vi "Request Multiple Data.vi"(4 "Ignore Past Updates? (F)":bool, 5 "Return Priority (Normal)":T2=enum."Normal", 6 "Value Changes Only? (T)":bool=TRUE, 7 "Activate Immediately? (T)":bool=TRUE, 8 "error in (no error)":errorcluster, 9 "Data Type":variant, 10 "Datum Names":string[](array[string]), 11 "IObserver in":refnum<class "IObserver.lvclass">) -> (0 "error out":errorcluster, 2 "Subscription Policies":T1[](array[typedef]), 3 "IObserver out":refnum<class "IObserver.lvclass">)   [LabVIEW 2015, in "IObserver.lvlib" / "IObserver.lvclass"]
doc: "<License>\nCopyright © 2017 Composed Systems, LLC | All rights reserved\nwww.composed.io\n\nAuthor: Ethan Stern <ethan.stern@composed.io>\n\nThis software is provided \"AS IS\" WITHOUT WARRANTIES, either express or implied, AND IS FOR EDUCATIONAL PURPOSES ONLY.\n</License>"
uses:
  IObserver.lvclass
  <vilib>/ActorFramework/Message Enqueuer/Message Priority.ctl
  IMediator/ISubscriptionPolicy/ISubscriptionPolicy Reference.ctl
  IMediator/ISubscriptionPolicy/ISubscriptionPolicy.lvclass
  <vilib>/ActorFramework/Message Enqueuer/Message Enqueuer.lvclass
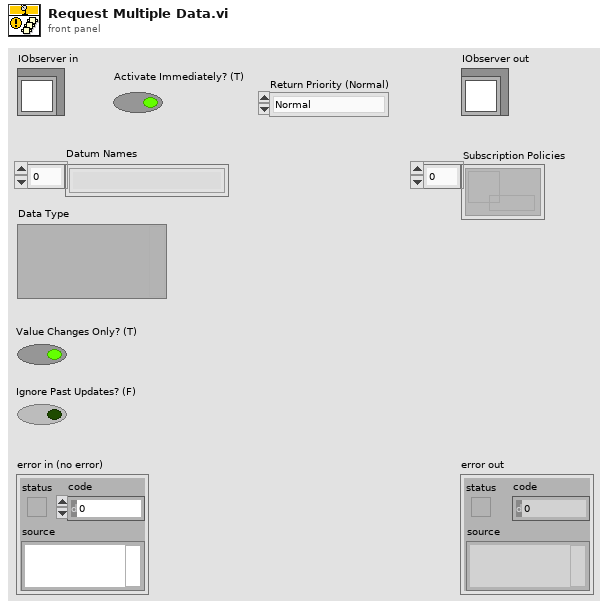
[diagram p1: front panel]
types:
  T1 = typedef "IMediator.lvlib/ISubscriptionPolicy.lvclass/ISubscriptionPolicy Reference.ctl" = refnum<data-value>
  T2 = typedef "Actor Framework.lvlib/Message Enqueuer.lvclass/Message Priority.ctl" = enum16{"Low", "Normal", "High"}
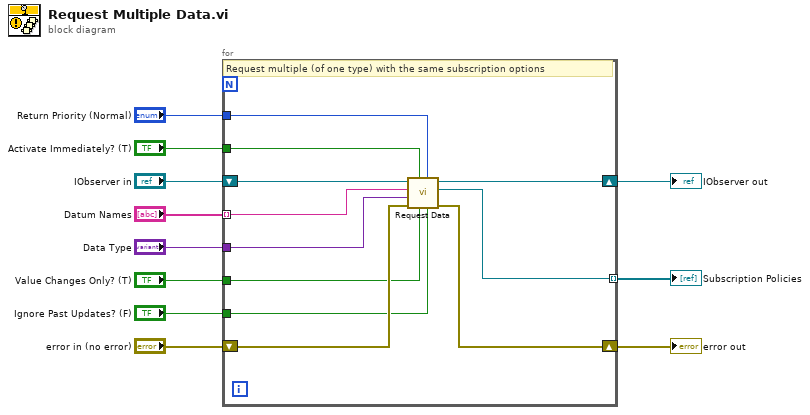
[diagram p0: block diagram]
diagram:
  n1 = for {
    shift-right: [w21] -> w10
    shift-left: "IObserver in" -> [w22]
    shift-right: [w19] -> w8
    shift-left: "error in (no error)" -> [w20]
    tunnel: [w18] -> w7 mode=indexing
    tunnel: "Datum Names" -> [w17] mode=indexing
    tunnel: "Data Type" -> [w16]
    tunnel: "Value Changes Only? (T)" -> [w15]
    tunnel: "Ignore Past Updates? (F)" -> [w14]
    tunnel: "Activate Immediately? (T)" -> [w13]
    tunnel: "Return Priority (Normal)" -> [w12]
    # "Request multiple (of one type) with the same subscription options"
    n2 = call "Request Data.vi"("Ignore Past Updates? (F)"=w14, "Return Priority (Normal)"=w12, "Value Changes Only? (T)"=w15, "Activate Immediately? (T)"=w13, "error in (no error)"=w20, "Data Type"=w16, "Datum Name"=w17, "IObserver in"=w22) -> ("error out"=w19:errorcluster, "Subscription Policy"=w18:T1, "IObserver out"=w21:refnum<class "IObserver.lvclass">)  [unwired: 1 in]
  }
  "error out" <- w8
  "IObserver out" <- w10
  "Subscription Policies" <- w7
